vi "GetChimeraResources.vi"(11 "Ring in":refnum<vi>) -> (3 "Array":string[](array[string]))   [LabVIEW 2025]
uses:
  <vilib>/nisyscfg/nisyscfg.lvlib
  <vilib>/nisyscfg/Filter Mode.ctl
  <resource>/objmgr/niflexrioatomicsae.rc
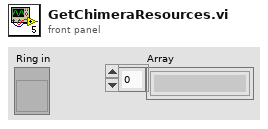
[diagram p1: front panel]
types:
  T1 = typedef "nisyscfg.lvlib/Filter Mode.ctl" = i32
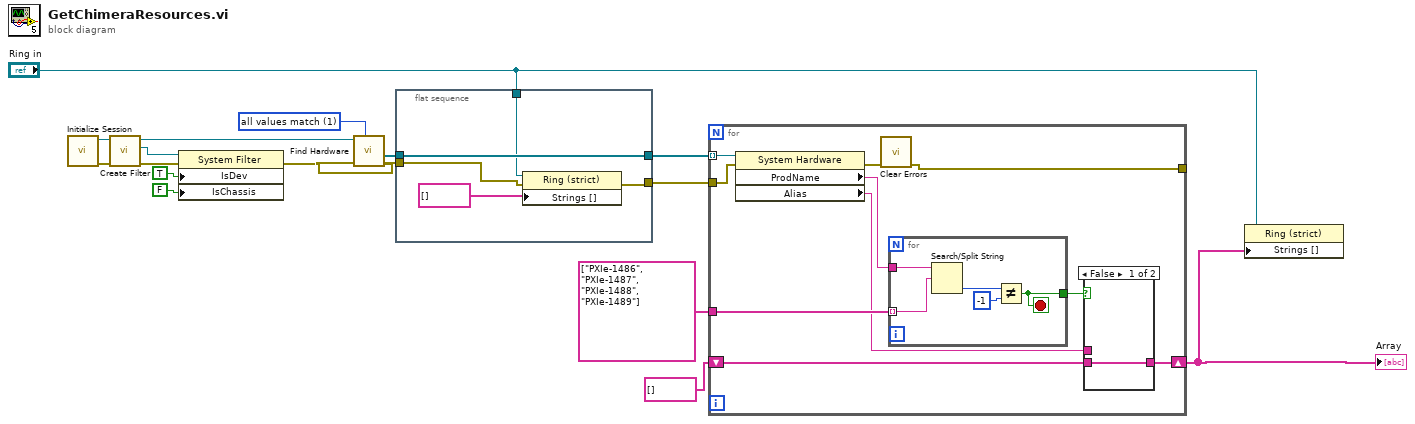
[diagram p0: block diagram]
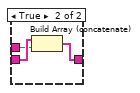
[diagram p2: hidden frame]
diagram:
  w2 = T1 1 items=["all values match"=1, "any value matches"=2, "values do not match"=3, "all properties exist"=4] ("Filter Mode (all values match)")
  n1 = call <vilib>:"Initialize Session.vi"() -> ("error out"=w5:errorcluster, "Session out"=w8:refnum<k21>)  [unwired: 10 in]
  n2 = call <vilib>:"Create Filter.vi"("error in (no error)"=w5, "Session in"=w8) -> ("error out"=w3:errorcluster, "Filter out"=w4:refnum<k20>, "Session out"=w9:refnum<k21>)  [unwired: 7 in]
  n3 = property class="System Filter"(reference=w4, error in=w3, "IsDev"=TRUE ("Is Chassis"), "IsChassis"=FALSE ("Is Chassis")) -> (error out=w13:errorcluster)  [unwired: 1 out]
  n4 = call <vilib>:"Find Hardware.vi"("Filter Mode (all values match)"=w2, "error in (no error)"=w13, "Session in"=w9) -> ("error out"=w14:errorcluster, "Resources out"=w12:refnum<k20>[])  [unwired: 5 in, 2 out]
  n5 = flat-sequence {
    tunnel: [w22] -> w1
    tunnel: w12 -> [w22]
    tunnel: w14 -> [w21]
    tunnel: [w19] -> w15
    tunnel: "Ring in" -> [w20]
    frame #0 {
      n6 = property class="Ring (strict)"(reference=w20, error in=w21, "Strings []"=string[] []) -> (error out=w19:errorcluster)  [unwired: 1 out]
    }
  }
  n7 = for {
    tunnel: w1 -> [w31] mode=indexing
    tunnel: string[] ["PXIe-1486", "PXIe-1487", "PXIe-1488", "PXIe-1489"] -> [w29]
    shift-right: [w28] -> w16
    shift-left: string[] [] -> [w27]
    tunnel: w15 -> [w24]
    tunnel: [w23] -> _
    n8 = property class="System Hardware"(reference=w31, error in=w24) -> (error out=w32:errorcluster, "ProdName"=w30:string, "Alias"=w25:string)  [unwired: 1 out]
    n9 = call <vilib>:"Clear Errors.vi"("error in (no error)"=w32) -> ("error out"=w23:errorcluster)  [unwired: 5 in, 1 out]
    n10 = for {
      tunnel: w30 -> [w41]
      tunnel: w29 -> [w40] mode=indexing
      tunnel: [w37] -> w26
      stop <- w37 stop-if-true
      n11 = Search/Split String(string=w41, search string/char (-)=w40) -> (offset of match=w39:i32)  [unwired: 1 in, 2 out]
      n12 = Not Equal?(x=w39, y=-1) -> (x != y?=w37:bool)
    }
    n13 = case shown="False" w26 {
      tunnel: [w33 w35] -> w28
      tunnel: w27 -> [w33 w36]
      tunnel: w25 -> [_ w34]
      frame False {
      }
      frame True {
        n14 = Build Array (concatenate)(w36, w34) -> (w35:string[])
      }
    }
  }
  "Array" <- w16
  n15 = property class="Ring (strict)"(reference="Ring in", "Strings []"=w16) -> ()  [unwired: 1 in, 2 out]
